vi "Get_Latest_Dust_Density.vi"(8 "error in (no error)":errorcluster, 11 "Small?":bool) -> (0 "error out":errorcluster, 3 "Density":dbl)   [LabVIEW 2013]
uses:
  <vilib>/addons/database/Connection.llb/Conn Execute.vi
  <vilib>/addons/database/Recordset.llb/Rec Fetch Recordset Data (R).vi
  <vilib>/addons/database/Recordset.llb/Rec Destroy - Connection.vi
  <vilib>/addons/database/_DB Variant To Data/Database Variant To Data.xnode
  <vilib>/addons/database/NI_Database_API.lvlib
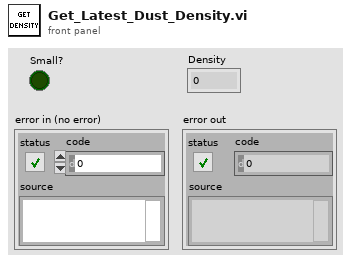
[diagram p1: front panel]
types:
  T1 = typedef "NI_Database_API.lvlib/Conn ObjectReference.ctl" = refnum<k1>
  T2 = typedef "NI_Database_API.lvlib/Rec ObjectReference.ctl" = refnum<k1>
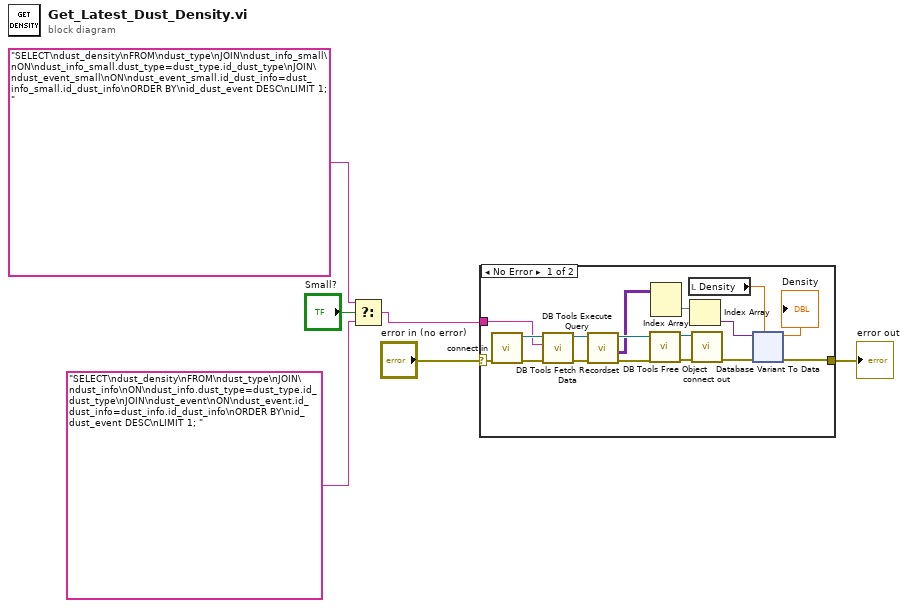
[diagram p0: block diagram]
diagram:
  n1 = Select(t="SELECT\ndust_density\nFROM\ndust_type\nJOIN\ndust_info_small\nON\ndust_info_small.dust_type=dust_type.id_dust_type\nJOIN\ndust_event_small\nON\ndust_event_small.id_dust_info=dust_info_small.id_dust_info\nORDER BY\nid_dust_event DESC\nLIMIT 1; ", s="Small?", f="SELECT\ndust_density\nFROM\ndust_type\nJOIN\ndust_info\nON\ndust_info.dust_type=dust_type.id_dust_type\nJOIN\ndust_event\nON\ndust_event.id_dust_info=dust_info.id_dust_info\nORDER BY\nid_dust_event DESC\nLIMIT 1; ") -> (s? t:f=w4:string)
  n2 = case shown="No Error" "error in (no error)" {
    selector: "error in (no error)" -> [w7 w56]
    tunnel: [w9 w56] -> w6
    tunnel: w4 -> [w8 _]
    frame No Error {
      n3 = call "connect in.vi"("error in (no error)"=w7) -> ("error out"=w23:errorcluster, "Database Connection"=w22:T1)  [unwired: 6 in, 1 out]
      n4 = call-poly <vilib>:"DB Tools Execute Query.vi"("error in (no error)"=w23, "SQL query"=w8, "connection reference"=w22) -> ("error out"=w21:errorcluster, "recordset reference"=w20:T2)  [unwired: 5 in]
      n5 = call-poly <vilib>:"DB Tools Fetch Recordset Data.vi"("error in (no error)"=w21, "recordset reference"=w20) -> ("error out"=w19:errorcluster, "recordset data"=w13:variant[][], "recordset reference out"=w18:T2)  [unwired: 3 in]
      n6 = call-poly <vilib>:"DB Tools Free Object.vi"("error in (no error)"=w19, "recordset reference"=w18) -> ("error out"=w16:errorcluster, "connection reference"=w17:T1)  [unwired: 8 in]
      n7 = Index Array(array=w13) -> (element=w12:variant[])  [unwired: 2 in]
      n8 = local read "Density"() -> (w10:dbl)
      n9 = Index Array(array=w12) -> (element=w11:variant)  [unwired: 1 in]
      n10 = call "connect out.vi"("error in (no error)"=w16, "connection reference"=w17) -> ("error out"=w14:errorcluster)  [unwired: 9 in]
      n11 = xnode "Database Variant To Data"("database variant"=w11, "error in (no error)"=w14, "type"=w10) -> ("data"=→"Density":dbl, "error out"=w9:errorcluster)
    }
    frame Error {
    }
  }
  "error out" <- w6
